vi "RT - Send Message to UI.vi"(8 "error in (no error)":errorcluster caption="错误输入（无错误）", 9 "Message Data":variant caption="消息数据", 10 "Message":string caption="消息") -> (0 "error out":errorcluster caption="错误输出")   [LabVIEW 2015]
uses:
  Message Queue/Message Cluster.ctl
  Globals/Global - Configuration Options.vi
  Globals/Global - RT Stream Connections.vi
  Message Queue/Message Queue.lvlib
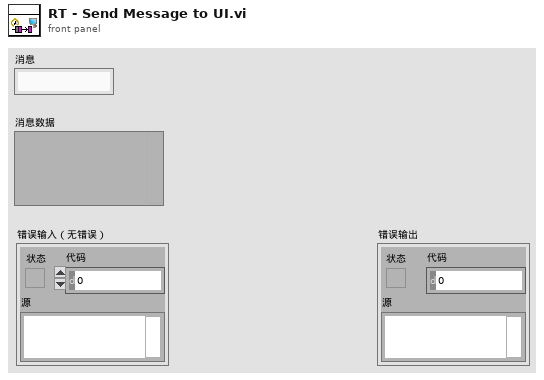
[diagram p1: front panel]
types:
  T1 = typedef "Message Queue.lvlib/Message Cluster.ctl" = cluster{"Message":string, "Message Data":variant}
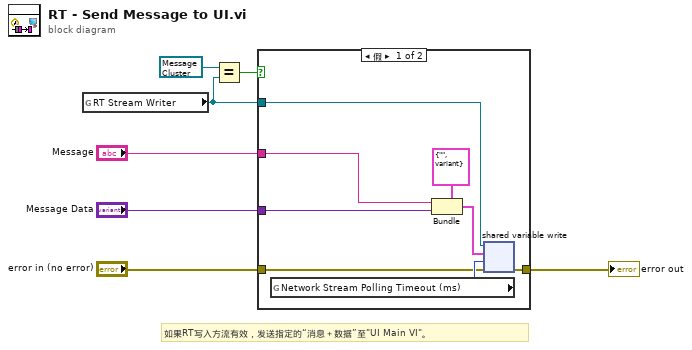
[diagram p0: block diagram]
diagram:
  # "如果RT写入方流有效，发送指定的“消息＋数据”至\"UI Main VI\"。"
  n1 = global read "Global - RT Stream Connections.vi" "RT Stream Writer"() -> (w5:refnum<k21>)
  n2 = Equal?(x=refnum<k21> refnum ("RT Writer Stream"), y=w5) -> (x = y?=w4:bool)
  n3 = case shown="假" w4 {
    tunnel: [w14 w16] -> w1
    tunnel: "error in (no error)" -> [w13 w16]
    tunnel: "Message Data" -> [w12 _]
    tunnel: w5 -> [w10 _]
    tunnel: "Message" -> [w8 _]
    frame False {
      n4 = global read "Global - Configuration Options.vi" "Network Stream Polling Timeout (ms)"() -> (w15:i32)
      n5 = Bundle(cluster=T1 {"Message"="", "Message Data"=variant} ("Message Cluster"), "Message"=w8, "Message Data"=w12) -> (w11:T1)
      n6 = shared-variable-write(w10, w13, w11, w15) -> (w14:errorcluster)  [unwired: 2 out]
    }
    frame True {
    }
  }
  "error out" <- w1
